vi "bind BLOB.vi"(8 "error in (no error)":errorcluster, 10 "String":string, 11 "SQLite3LV Cursor in":refnum<class "cursor.lvclass">) -> (0 "error out":errorcluster, 3 "SQLite3LV Cursor out":refnum<class "cursor.lvclass">)   [LabVIEW 2014, in "SQLite3LV.lvlib" / "cursor.lvclass"]
uses:
  cursor.lvclass
  cursor.lvclass/cursor.ctl
  SQLite3LV.lvlib
  sqlite3_64.dll
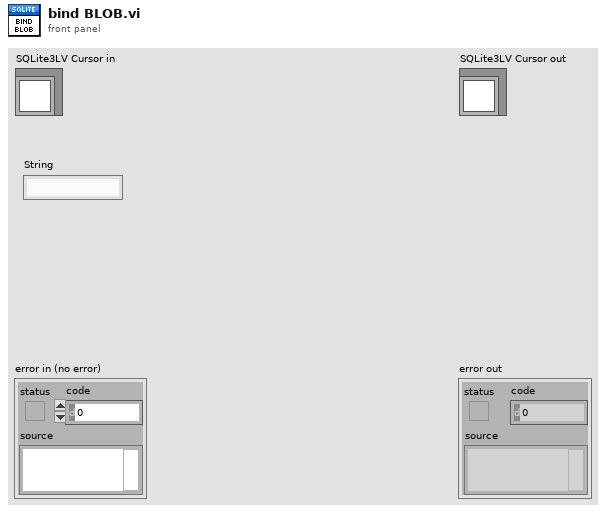
[diagram p1: front panel]
types:
  T1 = typedef "SQLite3LV.lvlib/cursor.lvclass/ctl_active_statement.ctl" = cluster{"ppStmt":i64, "column count":i32, "bind offset":i32, "bind param count":i32, "finished?":bool, "column offset":i32, "column types":i32[]}
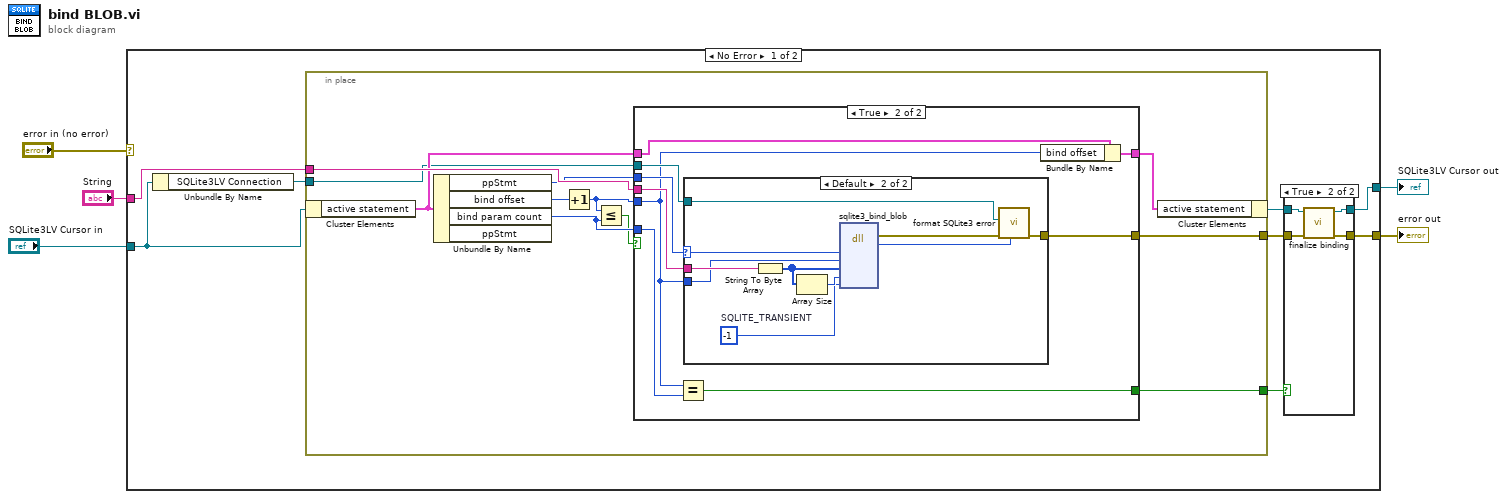
[diagram p0: block diagram]
diagram:
  n1 = case shown="No Error" "error in (no error)" {
    selector: "error in (no error)" -> [_ w52]
    tunnel: [w9 w52] -> w5
    tunnel: [w11 w51] -> w4
    tunnel: "SQLite3LV Cursor in" -> [w8 w51]
    tunnel: "String" -> [w13 _]
    frame No Error {
      n2 = Unbundle By Name(w8) -> ("SQLite3LV Connection"=w7:refnum<class "sqlite3.lvclass">)
      n3 = in-place {
        in-place-border: w13 -> [w30]
        in-place-border: [w29] -> w10
        in-place-border: w7 -> [w21]
        in-place-border: [w20] -> w6
        n4 = in-place-cluster #1(w8) -> ("active statement"=w23:T1)
        n5 = Unbundle By Name(w23) -> ("ppStmt"=w28:i64, "bind offset"=w27:i32, "bind param count"=w25:i32)  [unwired: 1 out]
        n6 = Increment(x=w27) -> (x+1=w26:i32)
        n7 = Less Or Equal?(x=w26, y=w25) -> (x <= y?=w24:bool)
        n8 = case shown="True" w24 {
          tunnel: w23 -> [w31 w40]
          tunnel: w30 -> [_ w39]
          tunnel: [w31 w38] -> w22
          tunnel: [_ w37] -> w29
          tunnel: w28 -> [_ w36]
          tunnel: w26 -> [_ w34]
          tunnel: w25 -> [_ w33]
          tunnel: w21 -> [_ w35]
          tunnel: [_ w32] -> w20
          frame False {
          }
          frame True {
            n9 = Equal?(x=w34, y=w33) -> (x = y?=w32:bool)
            n10 = case shown="Default" w36 {
              selector: w36 -> [_ w46]
              tunnel: [_ w50] -> w37
              tunnel: w34 -> [_ w47]
              tunnel: w39 -> [_ w48]
              tunnel: w35 -> [_ w42]
              frame 0 {
              }
              frame Default {
                w43 = i64 -1  # SQLITE_TRANSIENT
                n11 = String To Byte Array(string=w48) -> (unsigned byte array=w45:u8[])
                n12 = Array Size(array=w45) -> (size(s)=w44:i32)
                n13 = dll-call lib="C:/Users/BobUser/Desktop/LVTables/sqlite3**.*" fn="sqlite3_bind_blob"("pStmt"=w46, "index"=w47, "value"=w45, "nBytes"=w44, "pDestruct_NULL"=w43) -> (error out=w49:errorcluster, "column count"=w41:i32)  [unwired: 8 in, 1 out]
                n14 = call "format SQLite3 error.vi"("SQLite3LV Connection result"=w41, "error in (no error)"=w49, "psqlite"=w42) -> ("error out"=w50:errorcluster)  [unwired: 8 in]
              }
            }
            n15 = Bundle By Name(cluster=w40, "bind offset"=w34) -> (w38:T1)
          }
        }
        n16 = in-place-cluster #1("active statement"=w22) -> (w12:refnum<class "cursor.lvclass">)
      }
      n17 = case shown="True" w6 {
        tunnel: w12 -> [w15 w19]
        tunnel: [w15 w18] -> w11
        tunnel: w10 -> [w14 w17]
        tunnel: [w14 w16] -> w9
        frame False {
        }
        frame True {
          n18 = call "finalize binding.vi"("error in (no error)"=w17, "SQLite3LV Cursor in"=w19) -> ("error out"=w16:errorcluster, "SQLite3LV Cursor out"=w18:refnum<class "cursor.lvclass">)  [unwired: 8 in]
        }
      }
    }
    frame Error {
    }
  }
  "error out" <- w5
  "SQLite3LV Cursor out" <- w4
